vi "Open Report File.vi"(8 "error in (no error)":errorcluster, 11 "Coverage Report In":refnum<class "Coverage Report.lvclass">) -> (0 "error out":errorcluster, 3 "Coverage Report Out":refnum<class "Coverage Report.lvclass">)   [LabVIEW 2020, in "Coverage Report.lvclass"]
uses:
  Coverage Report.lvclass
  Coverage Report.lvclass/Coverage Report.ctl
  C:/git/astemes-lunit/source/Plugins/Coverage Report/Coverage Report.lvclass
  C:/git/astemes-lunit/source/Framework/Report Interface/Report Interface.lvclass
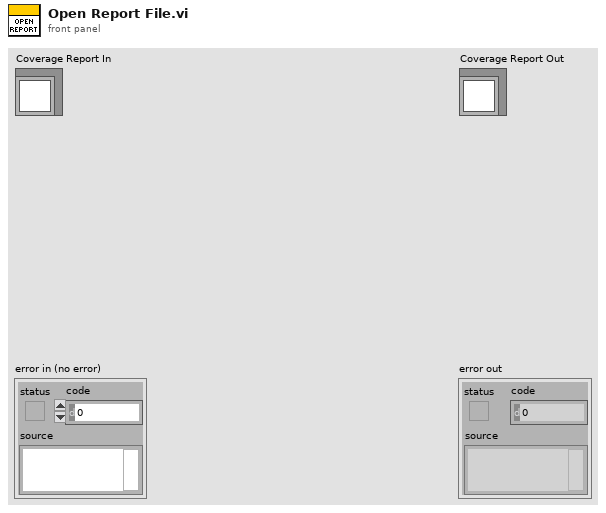
[diagram p1: front panel]
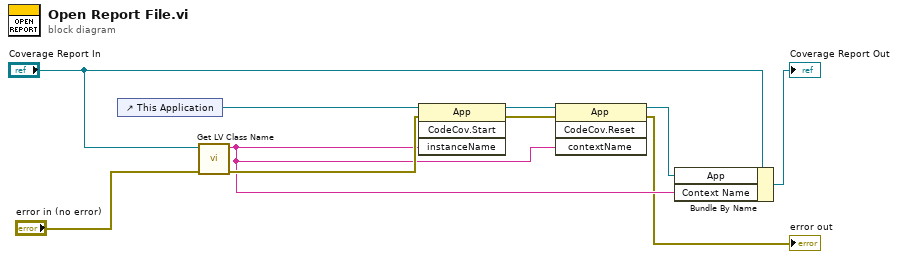
[diagram p0: block diagram]
diagram:
  n1 = control-ref of="This Application"() -> (w10:refnum<vi>)
  n2 = call <vilib>:"Get LV Class Name.vi"("error in (no error)"="error in (no error)", "object"="Coverage Report In") -> ("error out"=w5:errorcluster, "class name"=w4:string)  [unwired: 8 in]
  n3 = invoke class="App" method="CodeCov.Start"(reference=w10, error in=w5, "instanceName"=w4) -> (reference out=w8:refnum<vi>, error out=w9:errorcluster)  [unwired: 1 in, 2 out]
  n4 = invoke class="App" method="CodeCov.Reset"(reference=w8, error in=w9, "contextName"=w4) -> (reference out=w7:refnum<vi>, error out=→"error out":errorcluster)  [unwired: 1 in, 2 out]
  n5 = Bundle By Name(cluster="Coverage Report In", "App"=w7, "Context Name"=w4) -> (→"Coverage Report Out":refnum<class "Coverage Report.lvclass">)
